vi "Prepare Paths For Expiration Check.vi"(0 "SA Path Group in":refnum<class "SA Path Group.lvclass">, 5 "TSM Context":T1, 11 "error in":errorcluster) -> (4 "SA Path Group out":refnum<class "SA Path Group.lvclass">, 15 "error out":errorcluster)   [LabVIEW 2023, in "RFFixtureCharact.RMM.lvlib" / "SA Path Group.lvclass"]
uses:
  SA Path Group.lvclass
  C:/rfcal/AuxTools/STSRFFixtureCharactUtility/Source/Code Modules/Common/Base Classes/Path Group/Path Group.lvclass
  <vilib>/NI_TestStand_SemiconductorModule/NI_TestStand_Semiconductor_Module.lvlibp/PinMap/General/SemiconductorModuleContext.ctl
  Public/Charact Result Accessor/Scalar/Scalar Charact Result Accessor.lvclass
  C:/rfcal/AuxTools/STSRFFixtureCharactUtility/Source/Code Modules/Fixture/RMM/Charact Result Accessor/Base/Charact Result Accessor.lvclass
  C:/rfcal/AuxTools/STSRFFixtureCharactUtility/Source/Code Modules/Common/Result Accessor/Result Accessor.lvclass
  Common/Base Classes/Path/Path.lvclass/Path.ctl
  Common/Base Classes/Path/Properties/Read Interval.vi
  <vilib>/NI_TestStand_SemiconductorModule/NI_TestStand_Semiconductor_Module.lvlibp/PinMap/RF/RFmx/PinToNIRFmxSession.vi
  Common/Base Classes/Path/Path.lvclass
  SA Path Group.lvclass/SA Path Group.ctl
  <vilib>/NI_TestStand_SemiconductorModule/NI_TestStand_Semiconductor_Module.lvlibp
  Common/Base Classes/Path Group/Path Group.lvclass
  <vilib>/addons/_RFCalAndCharactDatabase/NI_RFCalAndCharact_Database_API.lvlibp/Characterization/Characterization.lvlib
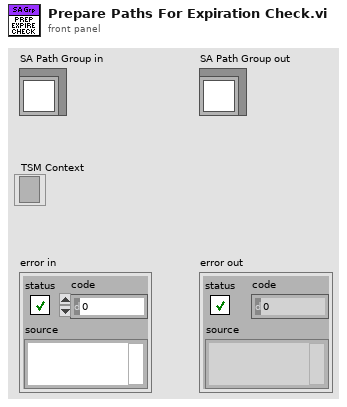
[diagram p1: front panel]
types:
  T1 = typedef "NI_TestStand_Semiconductor_Module.lvlibp/SemiconductorModuleContext.ctl" = refnum<k7>
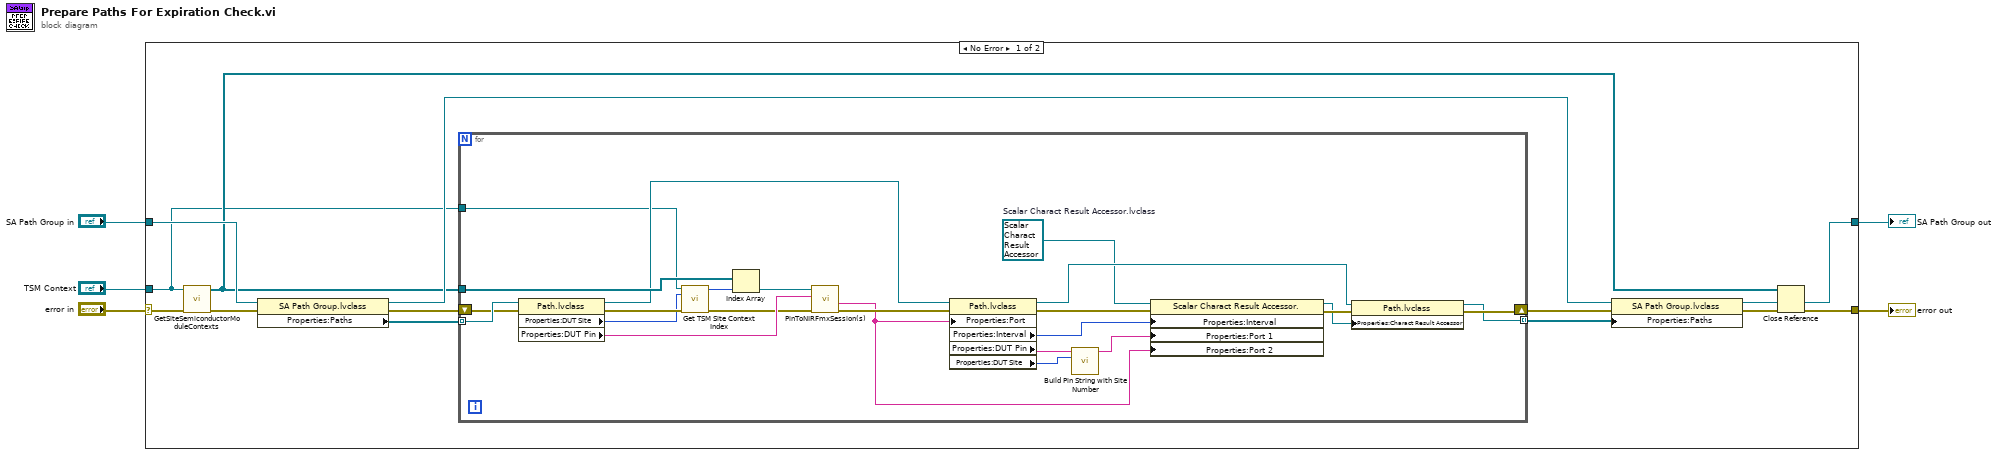
[diagram p0: block diagram]
diagram:
  n1 = case shown="No Error" "error in" {
    selector: "error in" -> [w10 w44]
    tunnel: "TSM Context" -> [w6 _]
    tunnel: "SA Path Group in" -> [w9 w43]
    tunnel: [w8 w44] -> w2
    tunnel: [w11 w43] -> w1
    frame No Error {
      n2 = call <vilib>:"GetSiteSemiconductorModuleContexts.vi"("error in (no error)"=w10, "Semiconductor Module Context"=w6) -> ("error out"=w15:errorcluster, "Site Semiconductor Module Contexts"=w7:T1[])  [unwired: 8 in]
      n3 = property class="SA Path Group.lvclass"(reference=w9, error in=w15) -> (reference out=w13:refnum<class "SA Path Group.lvclass">, error out=w17:errorcluster, "Properties:Paths"=w16:refnum<class "Path.lvclass">[])
      n4 = for {
        tunnel: w7 -> [w42]
        tunnel: w16 -> [w41] mode=indexing
        shift-right: [w27] -> w18
        shift-left: w17 -> [w39]
        tunnel: [w25] -> w12 mode=indexing
        tunnel: w6 -> [w33]
        w22 = refnum<class "Scalar Charact Result Accessor.lvclass"> refnum  # Scalar Charact Result Accessor.lvclass
        n5 = property class="Path.lvclass"(reference=w41, error in=w39) -> (reference out=w40:refnum<class "Path.lvclass">, error out=w38:errorcluster, "Properties:DUT Site"=w32:i32, "Properties:DUT Pin"=w36:string)
        n6 = call "Get TSM Site Context Index.vi"("Semiconductor Module Context"=w33, "Site Number"=w32, "error in (no error)"=w38) -> ("index of Site TSM Context"=w31:i32, "error out"=w34:errorcluster)  [unwired: 11 in]
        n7 = Index Array(array=w42, index=w31) -> (element=w37:T1)
        n8 = call-poly <vilib>:"PinToNIRFmxSession(s).vi"("error in (no error)"=w34, "Pin"=w36, "Semiconductor Module Context"=w37) -> ("error out"=w35:errorcluster, "Port"=w30:string)  [unwired: 4 in, 3 out]
        n9 = property class="Path.lvclass"(reference=w40, error in=w35, "Properties:Port"=w30) -> (reference out=w26:refnum<class "Path.lvclass">, error out=w21:errorcluster, "Properties:Interval"=w19:i32, "Properties:DUT Pin"=w24:string, "Properties:DUT Site"=w23:i32)
        n10 = call <vilib>:"Build Pin String with Site Number.vi"("Pin Name"=w24, "Site Number"=w23) -> ("Pin String"=w20:string)  [unwired: 13 in]
        n11 = property class="Scalar Charact Result Accessor."(reference=w22, error in=w21, "Properties:Interval"=w19, "Properties:Port 1"=w20, "Properties:Port 2"=w30) -> (reference out=w28:refnum<class "Scalar Charact Result Accessor.lvclass">, error out=w29:errorcluster)
        n12 = property class="Path.lvclass"(reference=w26, error in=w29, "Properties:Charact Result Accessor"=w28) -> (reference out=w25:refnum<class "Path.lvclass">, error out=w27:errorcluster)
      }
      n13 = property class="SA Path Group.lvclass"(reference=w13, error in=w18, "Properties:Paths"=w12) -> (reference out=w11:refnum<class "SA Path Group.lvclass">, error out=w14:errorcluster)
      n14 = Close Reference(reference=w7, error in (no error)=w14) -> (error out=w8:errorcluster)
    }
    frame Error {
    }
  }
  "error out" <- w2
  "SA Path Group out" <- w1
